vi "b2g_sqlite_write_feedflash.vi"(6 "Database File":string, 7 "feedflash.timestamp":timestamp, 8 "error in (no error)":errorcluster, 9 "Numeric":u64, 10 "seconds since 1Jan1904":timestamp, 11 "SQL Query":string) -> (0 "error out":errorcluster)   [LabVIEW 2011]
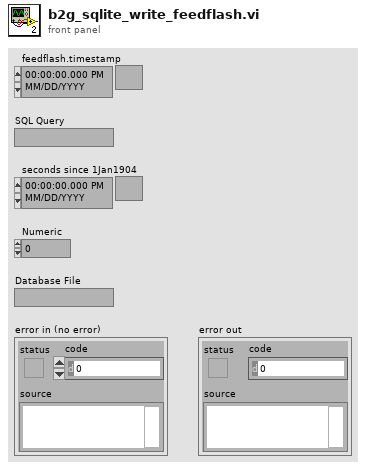
[diagram p1: front panel]
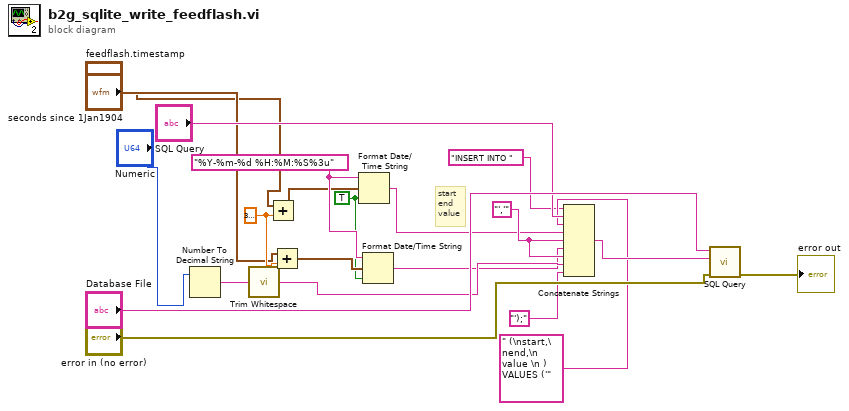
[diagram p0: block diagram]
diagram:
  w13 = "','" ("string")
  w4 = dbl[unit] 3600.0 ("y")
  w5 = TRUE ("UTC format")
  w7 = "%Y-%m-%d %H:%M:%S%3u" ("time format string (%c)")
  # "start\nend\nvalue"
  n1 = Number To Decimal String(number="Numeric") -> (decimal integer string=w8:string)  [unwired: 1 in]
  n2 = call <vilib>:"Trim Whitespace.vi"("string"=w8) -> ("trimmed string"=w12:string)  [unwired: 1 in]
  n3 = Add(x="feedflash.timestamp", y=w4) -> (x+y=w1:timestamp)
  n4 = Add(x="seconds since 1Jan1904", y=w4) -> (x+y=w6:timestamp)
  n5 = Format Date/Time String(time format string (%c)=w7, seconds (now)=w1, UTC format=w5) -> (date/time string=w10:string)
  n6 = Format Date/Time String(time format string (%c)=w7, seconds (now)=w6, UTC format=w5) -> (date/time string=w11:string)
  n7 = Concatenate Strings("INSERT INTO " ("SQL Query"), "SQL Query", " (\nstart,\nend,\n value \n ) VALUES ('" ("SQL Query"), w10, w13, w11, w13, w12, "');" ("string")) -> (w18:string)
  n8 = call "SQL Query.vi"("error in (no error)"="error in (no error)", "SQL Query"=w18, "Database File"="Database File") -> ("error out"=→"error out":errorcluster)  [unwired: 6 in, 2 out]
